vi "AG34980A_Initiate.vi"(0 "VISA resource name":refnum<visa-resource-name>, 11 "error in (no error)":errorcluster) -> (4 "VISA resource name out":refnum<visa-resource-name>, 15 "error out":errorcluster)   [LabVIEW 2022 SP3, in "DMM_Keysight_34980A.lvlib" / "DMM_Keysight_34980A.lvclass"]
doc: "This VI changes the state of the triggering system from the \"idle\" state to the \"wait-for-trigger\" state. Measurements will begin when the specified trigger conditions are satisfied following the receipt of the INITiate command issued by this VI. Note that this VI also clears the previous set of readings from memory."
uses:
  DMM_Keysight_34980A.lvclass
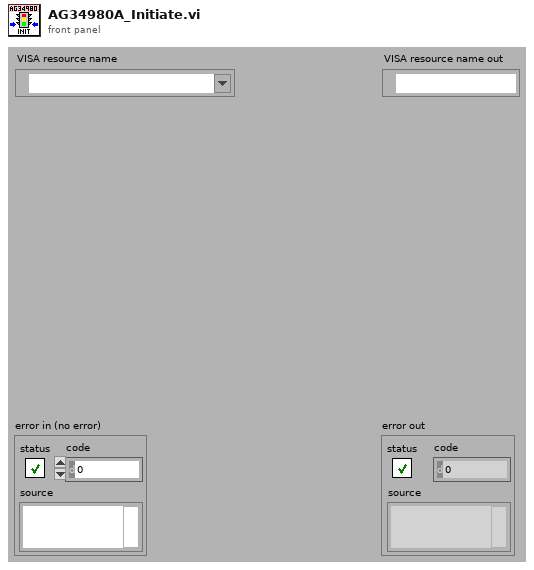
[diagram p1: front panel]
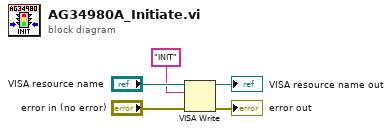
[diagram p0: block diagram]
diagram:
  n1 = VISA Write(VISA resource name="VISA resource name", write buffer="INIT", error in (no error)="error in (no error)") -> (VISA resource name out=→"VISA resource name out":refnum<visa-resource-name>, error out=→"error out":errorcluster)  [unwired: 1 out]
